vi "GetChildNodesBasedOnTag.vi"(10 "String":string, 11 "Child Nodes":cluster{"Type":string, "Node":variant}[](array[cluster])) -> (3 "Array":variant[](array[variant]))   [LabVIEW 2024]
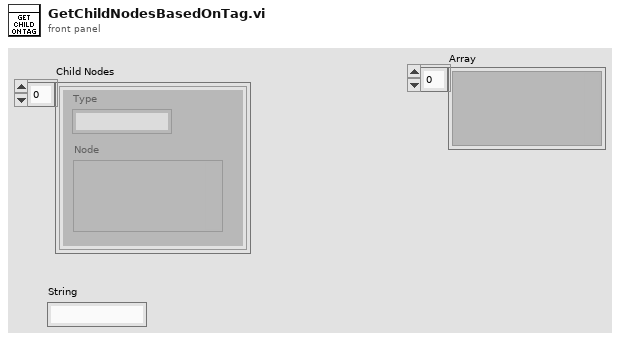
[diagram p1: front panel]
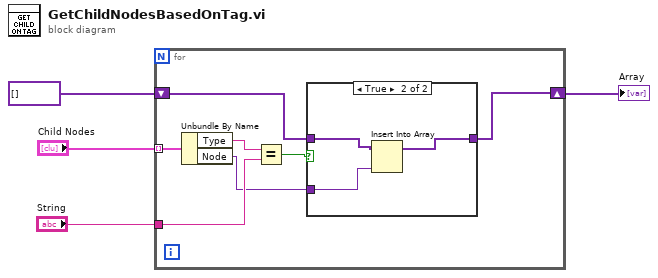
[diagram p0: block diagram]
diagram:
  n1 = for {
    tunnel: "Child Nodes" -> [w6] mode=indexing
    tunnel: "String" -> [w9]
    shift-right: [w7] -> w1
    shift-left: variant[] [] -> [w11]
    n2 = Unbundle By Name(w6) -> ("Type"=w10:string, "Node"=w5:variant)
    n3 = Equal?(x=w10, y=w9) -> (x = y?=w8:bool)
    n4 = case shown="True" w8 {
      tunnel: w11 -> [w12 w15]
      tunnel: [w12 w14] -> w7
      tunnel: w5 -> [_ w13]
      frame False {
      }
      frame True {
        n5 = Insert Into Array(array=w15, new element=w13) -> (w14:variant[])  [unwired: 1 in]
      }
    }
  }
  "Array" <- w1
